vi "SMC Global.vi"() -> ()   [LabVIEW 2010]
panel:
  in  "IPS Device":string
  in  "Witness Device":string
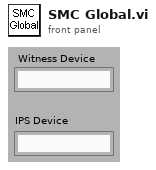
[diagram p1: front panel]
diagram:
